vi "drawEllipse.vi"(4 "ellipse in":dbl[](array[numeric])) -> (1 "XY ellipse":cluster{"x":dbl[], "y":dbl[]}(graph))   [LabVIEW 2014]
uses:
  <vilib>/imath/engines/lvmath2/RunTimeEngine/BuiltInFunctions/linramp/NIMS_linramp.vi
  <vilib>/imath/engines/lvmath2/RunTimeEngine/BuiltInFunctions/atan2/NIMS_atan2.vi
  <instcachedir>/0/NIMS_atan2_A91AA4A7D42247EDBE8F76DB99AF04A4.lvgen/NIMS_atan2_A91AA4A7D42247EDBE8F76DB99AF04A4_000.vi
  <vilib>/imath/engines/lvmath2/RunTimeEngine/ArithmeticOperatorToken/NIMS_ArithmeticOperator_minus.vi
  <instcachedir>/0/NIMS_ArithmeticOperator_minus_39C0593E74DA4138ACA2AB742906488D.lvgen/NIMS_ArithmeticOperator_minus_39C0593E74DA4138ACA2AB742906488D_000.vi
  <vilib>/imathl/engines/lvmath/Functions/Error Handling/Create Error.vi
  <vilib>/imath/engines/lvmath2/RunTimeEngine/ArithmeticOperatorToken/NIMS_ArithmeticOperator_plus.vi
  <instcachedir>/0/NIMS_ArithmeticOperator_plus_48D6EAACA5D645B09F7EC9C016C2DEA8.lvgen/NIMS_ArithmeticOperator_plus_48D6EAACA5D645B09F7EC9C016C2DEA8_001.vi
  <vilib>/imath/engines/lvmath2/RunTimeEngine/NodeEndStatement/NIMS_NodeEndStatement_Output.vi
  <instcachedir>/0/NIMS_NodeEndStatement_Output_53EC0D466D134D7ABD903AC30B43404B.lvgen/NIMS_NodeEndStatement_Output_53EC0D466D134D7ABD903AC30B43404B_000.vi
  <vilib>/imath/engines/lvmath2/RunTimeEngine/ErrorHandling/NIMS_Finalize Error.vi
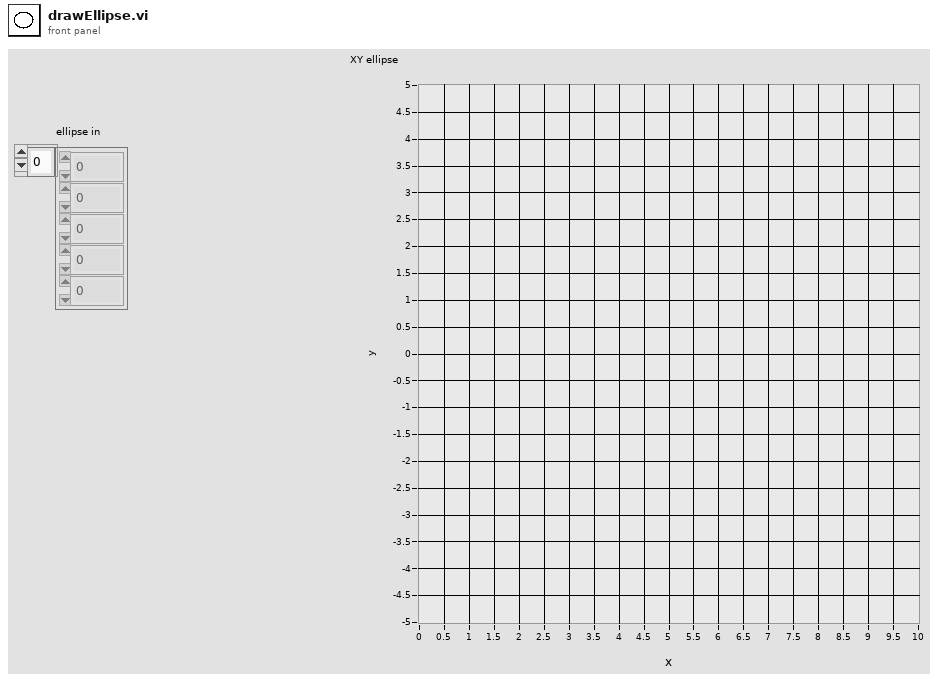
[diagram p1: front panel]
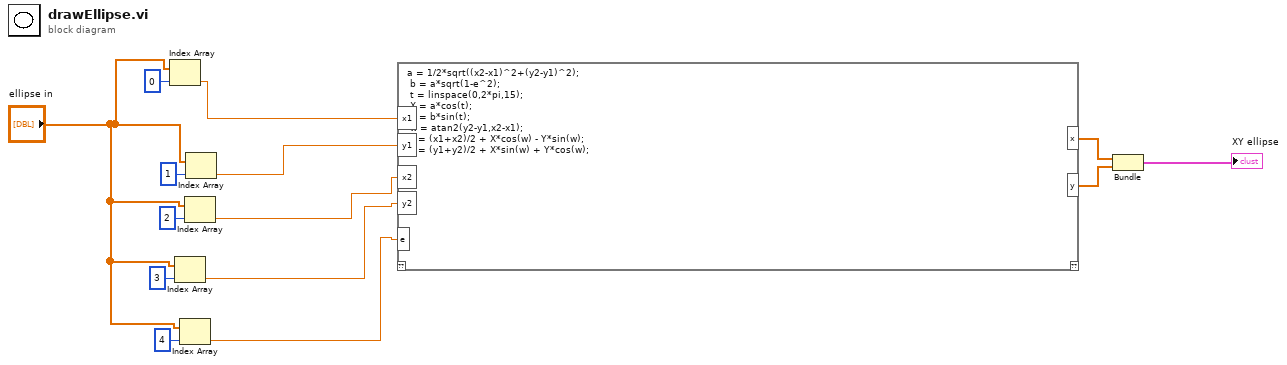
[diagram p0: block diagram]
diagram:
  n1 = Index Array(array="ellipse in", index=0) -> (element=w7:dbl)
  n2 = Index Array(array="ellipse in", index=3) -> (element=w4:dbl)
  n3 = Index Array(array="ellipse in", index=4) -> (element=w3:dbl)
  n4 = Index Array(array="ellipse in", index=2) -> (element=w5:dbl)
  n5 = Index Array(array="ellipse in", index=1) -> (element=w6:dbl)
  n6 = mathscript code="a = 1/2*sqrt((x2-x1)^2+(y2-y1)^2);\n b = a*sqrt(1-e^2);\n t = linspace(0,2*pi,15);\n X = a*cos(t);\n Y = b*sin(t);\n w = atan2(y2-y1,x2-x1);\n x = (x1+x2)/2 + X*cos(w) - Y*sin(w);\n y = (y1+y2)/2 + X*sin(w) + Y*cos(w);"("x1"=w7, "y1"=w6, "x2"=w5, "y2"=w4, "e"=w3) -> ("x"=w14:cdb[], "y"=w13:cdb[])  [unwired: 1 in, 1 out]
  n7 = Bundle("x"=w14, "y"=w13) -> (→"XY ellipse":cluster{"x":cdb[], "y":cdb[]})  [unwired: 1 in]
